vi "Commands 2 Cart Commands.vi"(10 "Cmd In":T1[](array[typedef])) -> (2 "Cart Commands Out":dbl[][](array[numeric]))   [LabVIEW 2009]
uses:
  Act & Cart Commands.ctl
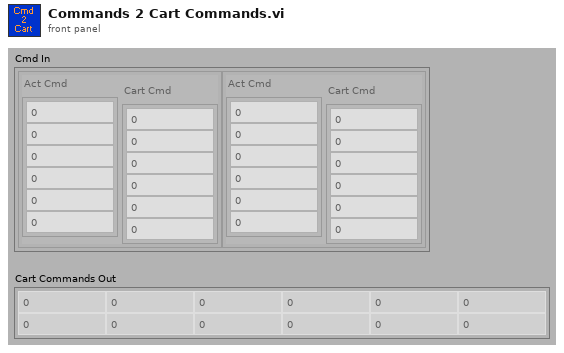
[diagram p1: front panel]
types:
  T1 = typedef "Act & Cart Commands.ctl" = cluster{"Act Cmd":dbl[], "Cart Cmd":dbl[]}
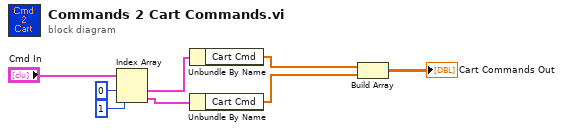
[diagram p0: block diagram]
diagram:
  n1 = Index Array(array="Cmd In", index #1=0 ("index"), index #2=1 ("index")) -> (element #1=w5:T1, element #2=w4:T1)
  n2 = Unbundle By Name(w5) -> ("Cart Cmd"=w3:dbl[])
  n3 = Unbundle By Name(w4) -> ("Cart Cmd"=w2:dbl[])
  n4 = Build Array(w3, w2) -> (→"Cart Commands Out":dbl[][])
